vi "LoadTabbedControls.vi"(8 "error in (no error)":errorcluster, 11 "VI in":refnum<vi>) -> (0 "error out":errorcluster, 3 "TabbedControls":T1[](array[typedef]))   [LabVIEW 2020, in "ContextHelpEditor.lvlib"]
uses:
  ContextHelpEditor.lvlib
  TabbedControl--cluster.ctl
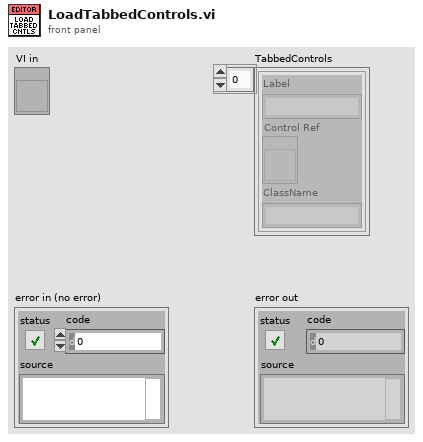
[diagram p1: front panel]
types:
  T1 = typedef "ContextHelpEditor.lvlib/TabbedControl--cluster.ctl" = cluster{"Label":string, "Control Ref":refnum<vi>, "ClassName":string}
  T2 = enum8{"Enabled", "Disabled", "Disabled and Grayed Out"}
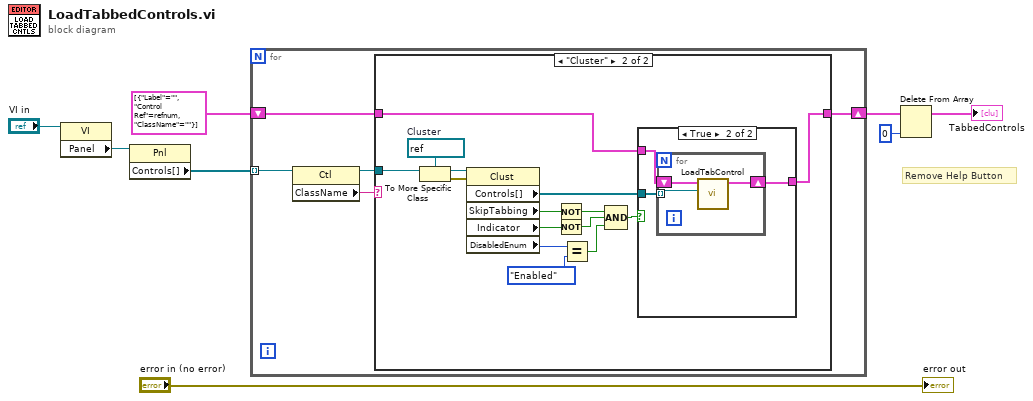
[diagram p0: block diagram]
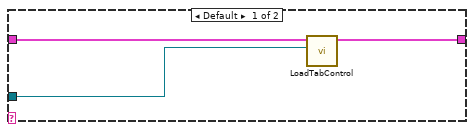
[diagram p2: hidden frame]
diagram:
  # "Remove Help Button"
  n1 = property class="VI"(reference="VI in") -> ("Panel"=w7:refnum<vi>)  [unwired: 1 in, 2 out]
  n2 = property class="Pnl"(reference=w7) -> ("Controls[]"=w6:refnum<vi>[])  [unwired: 1 in, 2 out]
  n3 = for {
    tunnel: w6 -> [w13] mode=indexing
    shift-right: [w9] -> w4
    shift-left: T1[] [{"Label"="", "Control Ref"=refnum, "ClassName"=""}] -> [w10]
    n4 = property class="Ctl"(reference=w13) -> (reference out=w11:refnum<vi>, "ClassName"=w12:string)  [unwired: 1 in, 1 out]
    n5 = case shown="\"Cluster\"" w12 {
      tunnel: w11 -> [w14 w31]
      tunnel: w10 -> [w15 w29]
      tunnel: [w16 w28] -> w9
      frame Default {
        n6 = call "LoadTabControl.vi"("Control in"=w14, "Array in"=w15) -> ("Array out"=w16:T1[])  [unwired: 9 in]
      }
      frame "Cluster" {
        w30 = refnum<vi> refnum  # Cluster
        n7 = To More Specific Class(target class=w30, reference=w31) -> (specific class reference=w20:refnum<vi>, error out=w17:errorcluster)  [unwired: 1 in]
        n8 = property class="Clust"(reference=w20, error in=w17) -> ("Controls[]"=w19:refnum<vi>[], "SkipTabbing"=w21:bool, "Indicator"=w22:bool, "DisabledEnum"=w23:T2)  [unwired: 2 out]
        n9 = Not(x=w21) -> (.not. x?=w25:bool)
        n10 = Not(x=w22) -> (.not. x?=w26:bool)
        n11 = Equal?(x=w23, y=T2."Enabled") -> (x = y?=w27:bool)
        n12 = Compound Arithmetic op=AND(w25, w26, w27) -> (w18:bool)
        n13 = case shown="True" w18 {
          tunnel: w29 -> [w32 w35]
          tunnel: [w32 w34] -> w28
          tunnel: w19 -> [_ w33]
          frame False {
          }
          frame True {
            n14 = for {
              tunnel: w33 -> [w38] mode=indexing
              shift-right: [w36] -> w34
              shift-left: w35 -> [w37]
              n15 = call "LoadTabControl.vi"("Control in"=w38, "Array in"=w37) -> ("Array out"=w36:T1[])  [unwired: 9 in]
            }
          }
        }
      }
    }
  }
  n16 = Delete From Array(array=w4, index=0) -> (array with subset deleted=→"TabbedControls":T1[])  [unwired: 1 in, 1 out]
  "error out" <- "error in (no error)"
